vi "SaveConfigFile.vi"(0 "IP":string caption="Robot IP Address", 1 "RoboguideRobotPath":path, 2 "ConnectRoboguide":bool, 3 "Use Telnet":bool, 4 "Telnet password":string, 5 "Use FTP":bool, 6 "FTP user":string, 7 "FTP password":string, 8 "Use SNPX":bool, 9 "error in (no error)":errorcluster, 10 "Licensee":string, 11 "Use CGTP":bool, 12 "Key":string, 13 "HTTP Login":string, 15 "HTTP Password":string caption="HTTP password") -> ()   [LabVIEW 2019]
uses:
  <vilib>/Utility/config.llb/NI_LVConfig.lvlib
  <vilib>/Utility/config.llb/Write Key (Path).vi
  <vilib>/Utility/config.llb/Write Key (String).vi
  <vilib>/Utility/config.llb/Write Key (Boolean).vi
panel:
  out "error out":errorcluster
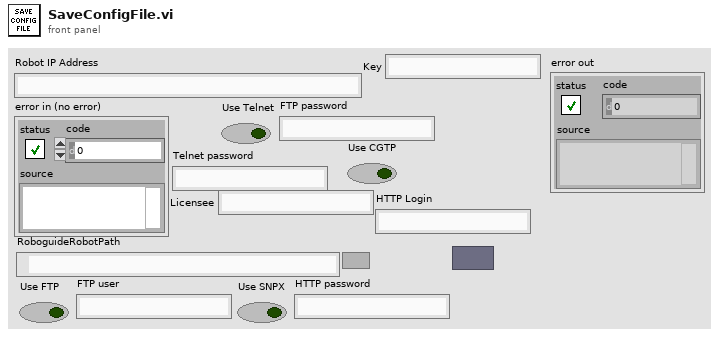
[diagram p1: front panel]
types:
  T1 = typedef "NI_LVConfig.lvlib/Config Data RefNum.ctl" = refnum<k1>
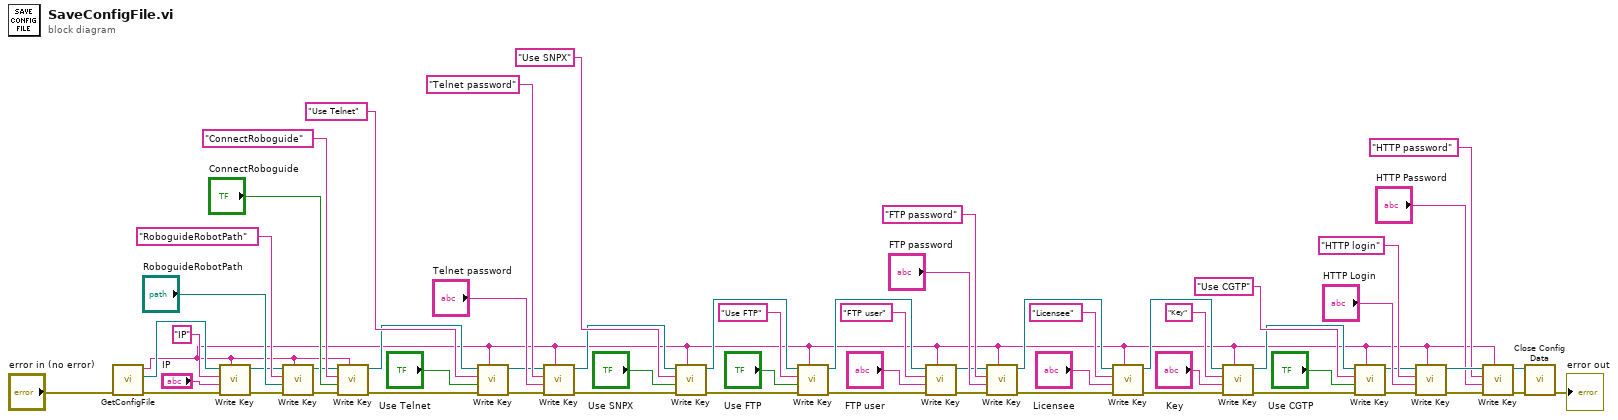
[diagram p0: block diagram]
diagram:
  n1 = call "GetConfigFile.vi"("error in (no error)"="error in (no error)") -> ("error out"=w60:errorcluster, "refnum"=w59:T1, "section"=w4:string)  [unwired: 8 in]
  n2 = call-poly <vilib>:"Write Key.vi"("section"=w4, "error in (no error)"=w60, "value"="IP", "key"="IP", "refnum"=w59) -> ("error out"=w28:errorcluster, "refnum out"=w16:T1)  [unwired: 4 in, 1 out]
  n3 = call-poly <vilib>:"Write Key.vi"("section"=w4, "error in (no error)"=w28, "value"="RoboguideRobotPath", "key"="RoboguideRobotPath", "refnum"=w16) -> ("error out"=w27:errorcluster, "refnum out"=w17:T1)  [unwired: 4 in, 1 out]
  n4 = call-poly <vilib>:"Write Key.vi"("section"=w4, "error in (no error)"=w27, "value"="ConnectRoboguide", "key"="ConnectRoboguide", "refnum"=w17) -> ("error out"=w26:errorcluster, "refnum out"=w29:T1)  [unwired: 4 in, 1 out]
  n5 = call-poly <vilib>:"Write Key.vi"("section"=w4, "error in (no error)"=w26, "value"="Use Telnet", "key"="Use Telnet", "refnum"=w29) -> ("error out"=w25:errorcluster, "refnum out"=w30:T1)  [unwired: 4 in, 1 out]
  n6 = call-poly <vilib>:"Write Key.vi"("section"=w4, "error in (no error)"=w25, "value"="Telnet password", "key"="Telnet password", "refnum"=w30) -> ("error out"=w24:errorcluster, "refnum out"=w31:T1)  [unwired: 4 in, 1 out]
  n7 = call-poly <vilib>:"Write Key.vi"("section"=w4, "error in (no error)"=w24, "value"="Use SNPX", "key"="Use SNPX", "refnum"=w31) -> ("error out"=w23:errorcluster, "refnum out"=w32:T1)  [unwired: 4 in, 1 out]
  n8 = call-poly <vilib>:"Write Key.vi"("section"=w4, "error in (no error)"=w23, "value"="Use FTP", "key"="Use FTP", "refnum"=w32) -> ("error out"=w22:errorcluster, "refnum out"=w33:T1)  [unwired: 4 in, 1 out]
  n9 = call-poly <vilib>:"Write Key.vi"("section"=w4, "error in (no error)"=w22, "value"="FTP user", "key"="FTP user", "refnum"=w33) -> ("error out"=w21:errorcluster, "refnum out"=w34:T1)  [unwired: 4 in, 1 out]
  n10 = call-poly <vilib>:"Write Key.vi"("section"=w4, "error in (no error)"=w21, "value"="FTP password", "key"="FTP password", "refnum"=w34) -> ("error out"=w20:errorcluster, "refnum out"=w35:T1)  [unwired: 4 in, 1 out]
  n11 = call-poly <vilib>:"Write Key.vi"("section"=w4, "error in (no error)"=w20, "value"="Licensee", "key"="Licensee", "refnum"=w35) -> ("error out"=w19:errorcluster, "refnum out"=w36:T1)  [unwired: 4 in, 1 out]
  n12 = call-poly <vilib>:"Write Key.vi"("section"=w4, "error in (no error)"=w19, "value"="Key", "key"="Key", "refnum"=w36) -> ("error out"=w13:errorcluster, "refnum out"=w12:T1)  [unwired: 4 in, 1 out]
  n13 = call-poly <vilib>:"Write Key.vi"("section"=w4, "error in (no error)"=w13, "value"="Use CGTP", "key"="Use CGTP", "refnum"=w12) -> ("error out"=w5:errorcluster, "refnum out"=w3:T1)  [unwired: 4 in, 1 out]
  n14 = call-poly <vilib>:"Write Key.vi"("section"=w4, "error in (no error)"=w5, "value"="HTTP Login", "key"="HTTP login", "refnum"=w3) -> ("error out"=w11:errorcluster, "refnum out"=w10:T1)  [unwired: 4 in, 1 out]
  n15 = call-poly <vilib>:"Write Key.vi"("section"=w4, "error in (no error)"=w11, "value"="HTTP Password", "key"="HTTP password", "refnum"=w10) -> ("error out"=w2:errorcluster, "refnum out"=w1:T1)  [unwired: 4 in, 1 out]
  n16 = call <vilib>:"Close Config Data.vi"("error in (no error)"=w2, "refnum"=w1) -> ("error out"=→"error out":errorcluster)  [unwired: 8 in, 1 out]
